vi "mm2time.vi"(2 "Offset (mm)":dbl, 3 "distance (mm)":dbl) -> (0 "time in fs":dbl)   [LabVIEW 2020]
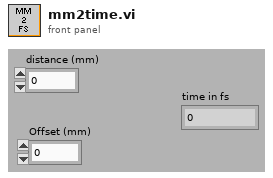
[diagram p1: front panel]
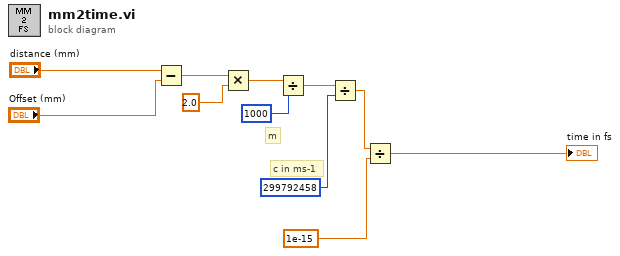
[diagram p0: block diagram]
diagram:
  # "c in ms-1"
  # "m"
  n1 = Subtract(x="distance (mm)", y="Offset (mm)") -> (x-y=w3:dbl)
  n2 = Multiply(x=w3, y=2.0) -> (x*y=w5:dbl)
  n3 = Divide(x=w5, y=1000) -> (x/y=w7:dbl)
  n4 = Divide(x=w7, y=299792458) -> (x/y=w2:dbl)
  n5 = Divide(x=w2, y=1e-15) -> (x/y=→"time in fs":dbl)
